vi "Init_Instr.vi"(8 "error in (no error)":errorcluster caption="entrée d'erreur (pas d'erreur)", 11 "Class Relay_Board en entrée":refnum<class "Class Instrument Relay_Board.lvclass">) -> (0 "error out":errorcluster caption="sortie d'erreur", 3 "Class Relay_Board en Sortie":refnum<class "Class Instrument Relay_Board.lvclass">)   [LabVIEW 2020, in "Library Instrument & Equipement.lvlib" / "Library Instruments.lvlib" / "Class Instrument Relay_Board.lvclass"]
uses:
  Class Instrument Relay_Board.lvclass
  Class Instrument Relay_Board.lvclass/Class Instrument Relay_Board.ctl
  Instrument (Default)/Class Instrument (Default).lvclass
  Relay_Board/Relay_Board (Default)/Class Relay_Board (Default).lvclass
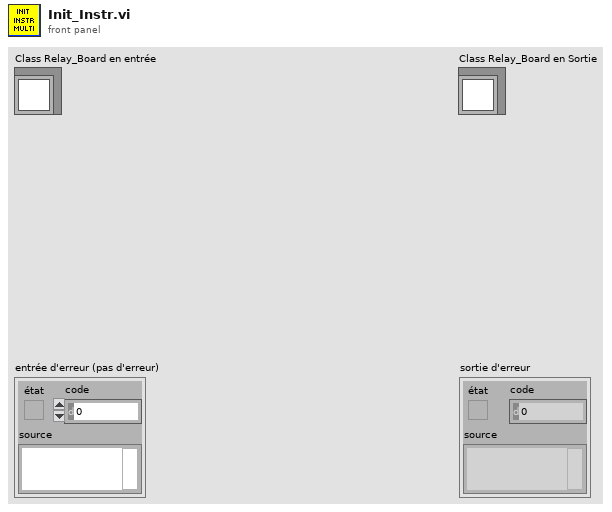
[diagram p1: front panel]
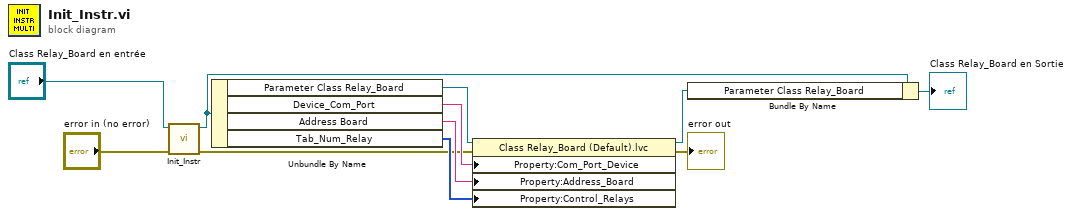
[diagram p0: block diagram]
diagram:
  n1 = call-parent "Init_Instr.vi"("error in (no error)"="error in (no error)", "Class Instrument (Default) en entrée"="Class Relay_Board en entrée") -> ("error out"=w5:errorcluster, "Class Instrument (Default) en sortie"=w3:refnum<class "Class Instrument Relay_Board.lvclass">)  [unwired: 8 in]
  n2 = Unbundle By Name(w3) -> ("Parameter Class Relay_Board"=w9:refnum<class "Class Relay_Board (Default).lvclass">, "Device_Com_Port"=w8:string, "Address Board"=w7:string, "Tab_Num_Relay"=w6:u8[])
  n3 = property class="Class Relay_Board (Default).lvc"(reference=w9, error in=w5, "Property:Com_Port_Device"=w8, "Property:Address_Board"=w7, "Property:Control_Relays"=w6) -> (reference out=w1:refnum<class "Class Relay_Board (Default).lvclass">, error out=→"error out":errorcluster)
  n4 = Bundle By Name(cluster=w3, "Parameter Class Relay_Board"=w1) -> (→"Class Relay_Board en Sortie":refnum<class "Class Instrument Relay_Board.lvclass">)
